vi "Peak.vi"(0 "2d Data":sgl[][](array[numeric]) format="%0.3f", 1 "Fitting Function":string(combo)="lorentz", 2 "Visible":i32(ring) items=["MAINWND_HIDE"=0, "MAINWND_SHOW"=1, "MAINWND_SHOWMINIMIZED"=2, "MAINWND_SHOWMAXIMIZED"=3, "MAINWND_SHOW_BRING_TO_FRONT"=100]) -> (3 "Peak Center":dbl format="%#_9g", 4 "Peak Width":dbl, 5 "Peak Height":dbl, 6 "Fit":cluster{"data":dbl[], "data":dbl[]}[](graph))   [LabVIEW 2014]
panel:
  in  "ogw path":path=path "E:/LabVIEW/Include/iontrap.net.llb/Peak.ogw"
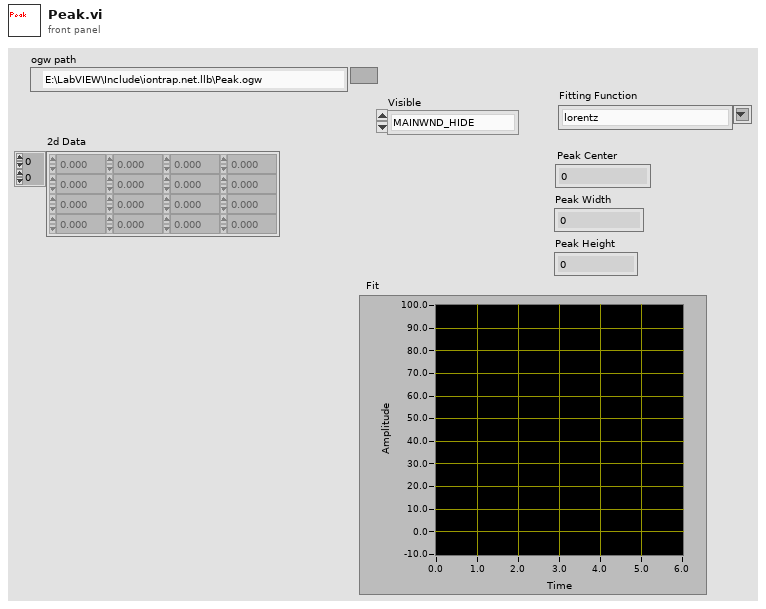
[diagram p1: front panel]
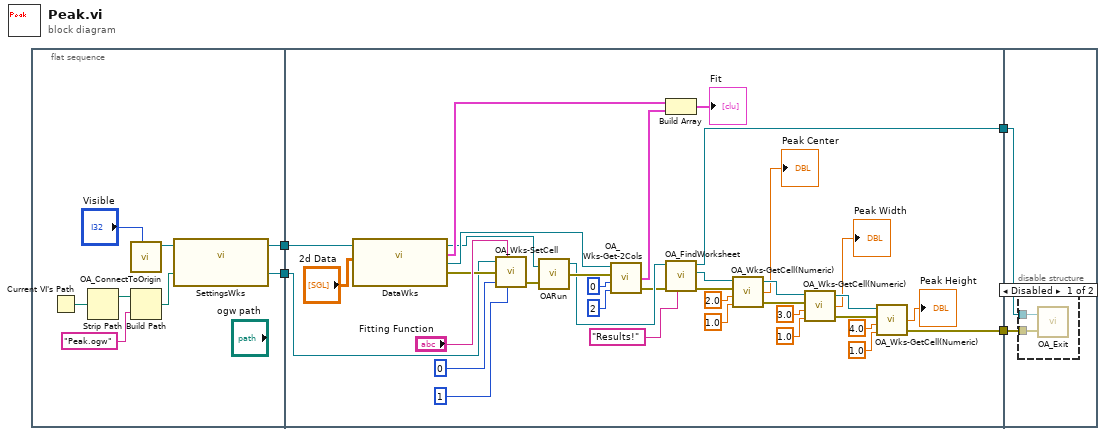
[diagram p0: block diagram]
diagram:
  n1 = flat-sequence {
    tunnel: [w11] -> w2
    tunnel: [w10] -> w1
    tunnel: w2 -> [w16]
    tunnel: w1 -> [w15]
    tunnel: [w14] -> w4
    tunnel: [w13] -> w3
    tunnel: w4 -> [w50]
    tunnel: w3 -> [w49]
    frame #0 {
      n2 = Current VI's Path() -> (path=w8:path)
      n3 = Strip Path(path=w8) -> (stripped path=w7:path)  [unwired: 1 out]
      n4 = call <userlib>:"OA_ConnectToOrigin.vi"("Visible"="Visible") -> ("Origin.IOApplication"=w12:refnum<k7>)  [unwired: 7 in, 1 out]
      n5 = Build Path(base path=w7, name or relative path="Peak.ogw") -> (appended path=w5:path)
      n6 = call "SettingsWks.vi"("Path"=w5, "Origin.IOApplication"=w12) -> ("SettingsWks"=w10:refnum<k7>, "Origin.IOApplication"=w11:refnum<k7>)
    }
    frame #1 {
      n7 = call "DataWks.vi"("Origin.IOApplication"=w16, "2d Data"="2d Data") -> ("Origin.IOApplication"=w18:refnum<k7>, "Input Data"=w20:cluster{"data":dbl[], "data":dbl[]}, "DataWks"=w23:refnum<k7>, "error out"=w22:errorcluster)  [unwired: 1 in]
      n8 = call <vilib>:"OA_Wks-SetCell.vi"("Origin.Worksheet"=w15, "Data"="Fitting Function", "error in (no error)"=w22, "r1"=0, "c1"=1) -> ("error out"=w45:errorcluster)  [unwired: 2 out]
      n9 = call <vilib>:"OARun.vi"("Origin.IOApplication"=w18, "Error IO"=w45) -> ("Origin.IOApplication"=w41:refnum<k7>, "Error IO Out"=w42:errorcluster)  [unwired: 1 out]
      n10 = call <vilib>:"OA_Wks-Get-2Cols.vi"("yCol"=2, "xCol"=0, "error in (no error)"=w42, "Origin.Worksheet"=w23) -> ("error out"=w40:errorcluster, "Bundled Cols"=w19:cluster{"data":dbl[], "data":dbl[]})  [unwired: 1 out]
      n11 = Build Array(w20, w19) -> (→"Fit":cluster{"data":dbl[], "data":dbl[]}[])
      n12 = call <vilib>:"OA_FindWorksheet.vi"("Name"="Results!", "error in (no error)"=w40, "Origin.IOApplication"=w41) -> ("error out"=w37:errorcluster, "Origin.Worksheet"=w38:refnum<k7>, "Origin.IOApplication"=w14:refnum<k7>)  [unwired: 6 in]
      n13 = call <vilib>:"OA_Wks-GetCell(Numeric).vi"("c1"=1.0, "r1"=2.0, "error in (no error)"=w37, "Origin.Worksheet"=w38) -> ("error out"=w31:errorcluster, "Data"=→"Peak Center":dbl, "Origin.Worksheet Out"=w32:refnum<k7>)
      n14 = call <vilib>:"OA_Wks-GetCell(Numeric).vi"("c1"=1.0, "r1"=3.0, "error in (no error)"=w31, "Origin.Worksheet"=w32) -> ("error out"=w28:errorcluster, "Data"=→"Peak Width":dbl, "Origin.Worksheet Out"=w29:refnum<k7>)
      n15 = call <vilib>:"OA_Wks-GetCell(Numeric).vi"("c1"=1.0, "r1"=4.0, "error in (no error)"=w28, "Origin.Worksheet"=w29) -> ("error out"=w13:errorcluster, "Data"=→"Peak Height":dbl)  [unwired: 1 out]
    }
    frame #2 {
      n16 = disable-structure shown="Disabled" {
        disable-tunnel: w50 -> [w52 _]
        disable-tunnel: w49 -> [w51 _]
        frame Disabled {
          n17 = call <userlib>:"OA_Exit.vi"("Error IO"=w51, "Origin.IOApplication"=w52) -> ()  [unwired: 2 out]
        }
        frame Enabled {
        }
      }
    }
  }
